vi "acquireAndDetectTest.vi"() -> ()   [LabVIEW 2024]
uses:
  src/elements/black-squircle-dropdown.ctl
  src/toolkit/modelParameters.ctl
  src/elements/black-squircle-ring.ctl
  <vilib>/Utility/error.llb/DialogType.ctl
  <vilib>/vision/driver/NI_Vision_Acquisition_Software.lvlib
  <resource>/objmgr/imaqdx.rc
  src/toolkit/transformCvToolkit.lvclass
panel:
  out "error status":string
  in  "update model":bool
  in  "res":T1 caption="Resolution:" items=["160x120 YUY2 30.00fps", "320x180 YUY2 30.00fps", "320x240 YUY2 30.00fps", "424x240 YUY2 30.00fps", "640x360 MJPG 30.00fps", "640x360 YUY2 30.00fps", "640x480 MJPG 30.00fps", "640x480 YUY2 30.00fps", "848x480 MJPG 30.00fps", "960x540 MJPG 30.00fps", "1280x720 MJPG 30.00fps"]
  in  "pause":bool
  in  "model params":T2={"conf"=0.25, "iou"=0.5, "model w"=1280, "model h"=736, "img w "=1280, "img h"=736} caption="Model Parameters"
  in  "classes":path caption="Class Definition Path"
  in  "model":path caption="Model Path"
  in  "cpu/gpu":enum32{"Item 0", "Item 1"}(radio)=enum."Item 1"
  in  "play":bool
  in  "cam":T3 caption="Camera:"
  out "img":T4(plugin-control)
  out "tot detect":i32 caption="Total Detections"
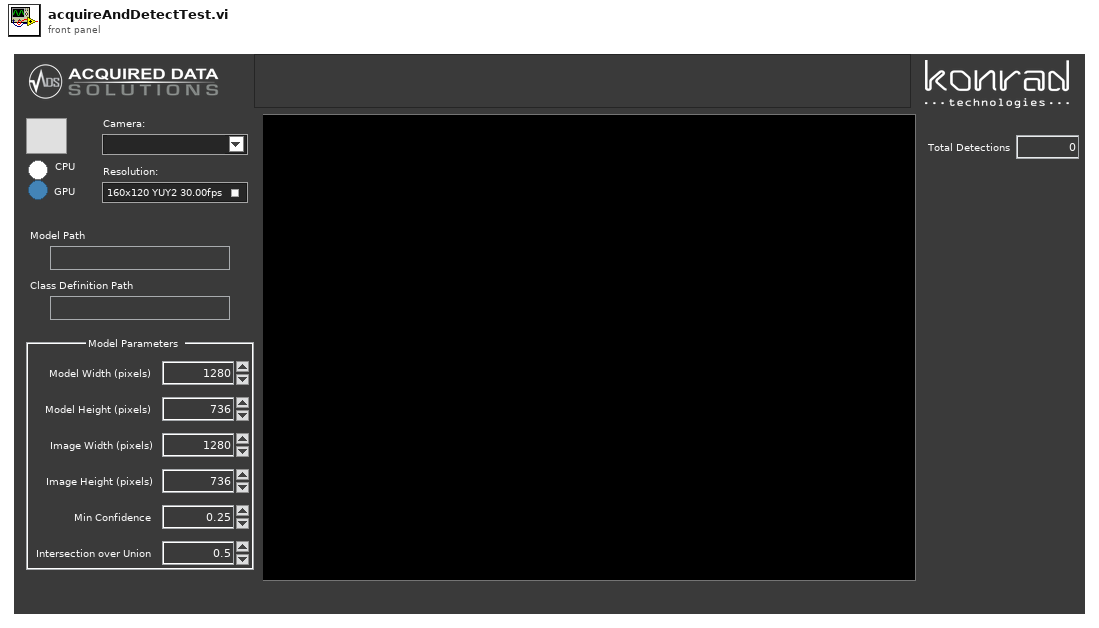
[diagram p1: front panel]
types:
  T1 = typedef "black-squircle-ring.ctl" = u16
  T2 = typedef "transformCvToolkit.lvclass/modelParameters.ctl" = cluster{"conf":dbl, "iou":dbl, "model w":i32, "model h":i32, "img w ":i32, "img h":i32}
  T3 = typedef "black-squircle-dropdown.ctl" = string
  T4 = typedef "IMAQ Image.ctl" = refnum<image>
  T5 = typedef "IMAQdx.ctl" = refnum<k21>
  T6 = typedef "DialogType.ctl" = u16
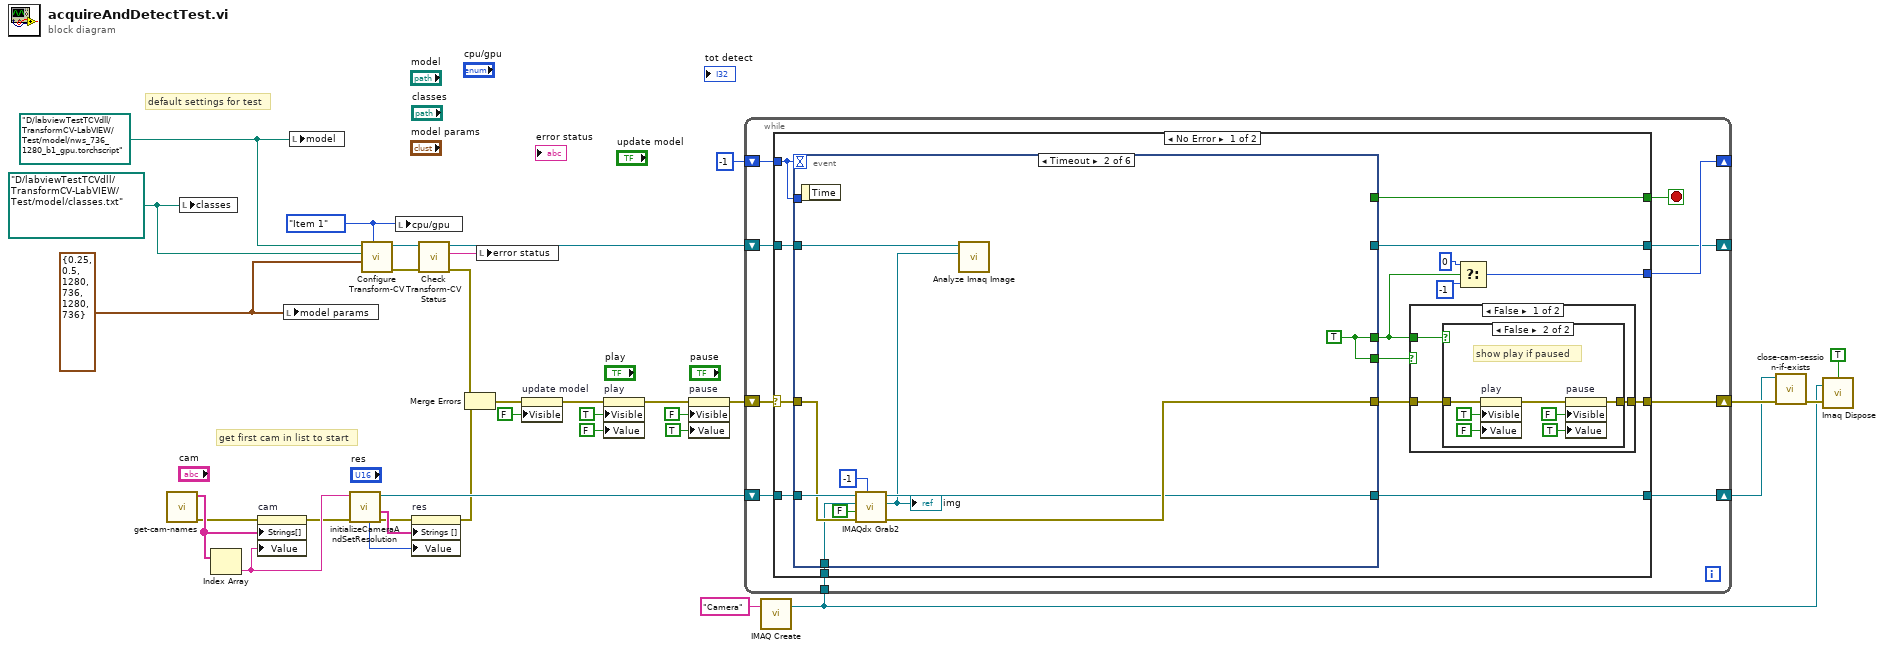
[diagram p0: block diagram]
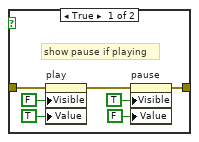
[diagram p2: hidden frame]
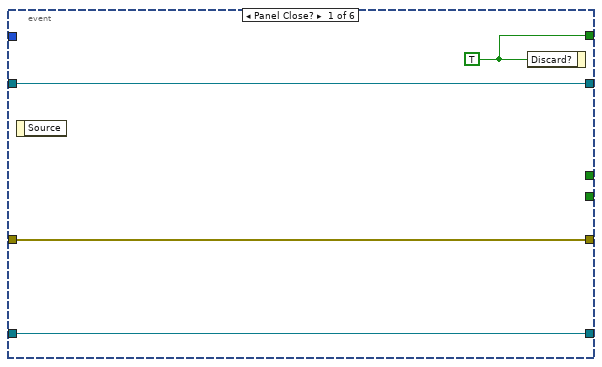
[diagram p4: hidden frame]
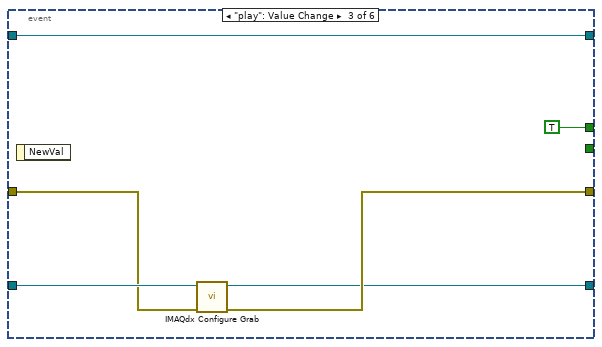
[diagram p5: hidden frame]
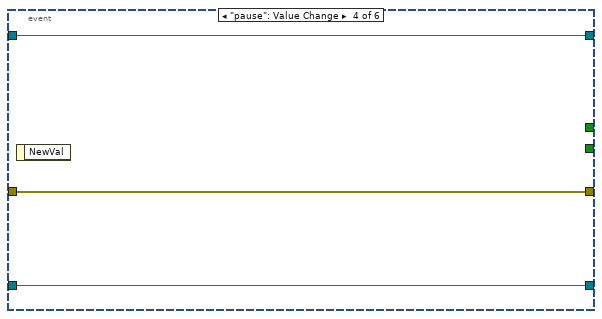
[diagram p6: hidden frame]
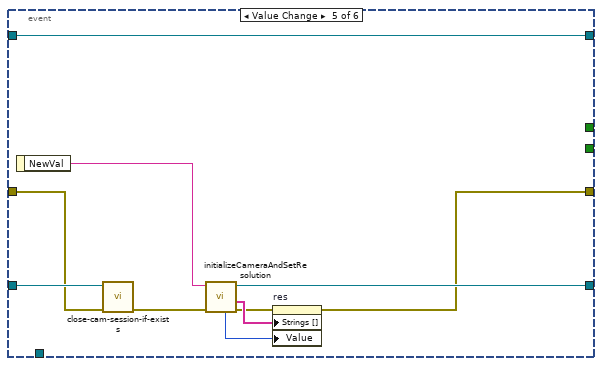
[diagram p7: hidden frame]
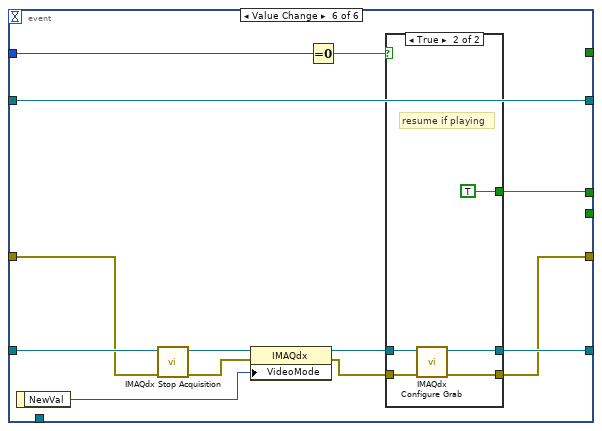
[diagram p8: hidden frame]
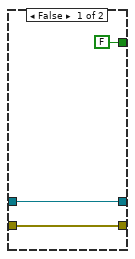
[diagram p9: hidden frame]
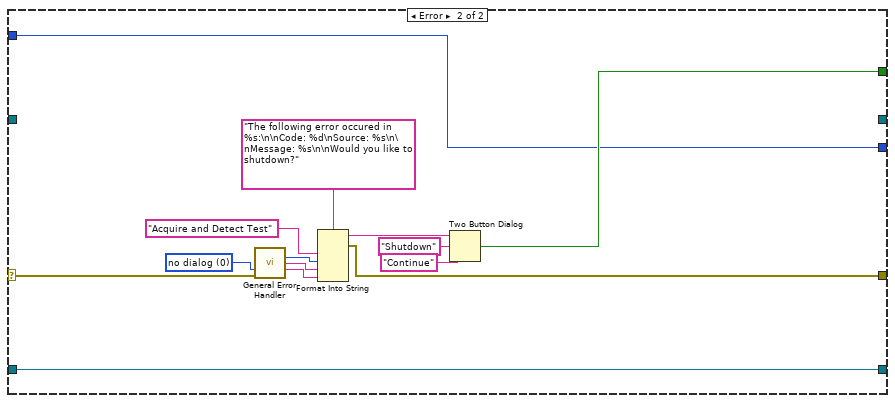
[diagram p10: hidden frame]
diagram:
  w6 = enum32{"Item 0", "Item 1"}."Item 1" ("cpu/gpu")
  w9 = T2 {"conf"=0.25, "iou"=0.5, "model w"=1280, "model h"=736, "img w "=1280, "img h"=736} ("model params")
  w10 = path "D:/labviewTestTCVdll/TransformCV-LabVIEW/Test/model/classes.txt" ("model")
  w11 = path "D:/labviewTestTCVdll/TransformCV-LabVIEW/Test/model/nws_736_1280_b1_gpu.torchscript" ("model")
  # "get first cam in list to start"
  # "default settings for test"
  n1 = call "get-cam-names.vi"() -> ("error out"=w12:errorcluster, "cam names"=w27:string[])  [unwired: 10 in]
  n2 = local write "classes"(w10) -> ()
  n3 = Index Array(array=w27) -> (element=w26:string)  [unwired: 1 in]
  n4 = property on="cam" class="CmbBox (strict)"(error in=w12, "Strings[]"=w27, "Value"=w26) -> (error out=w25:errorcluster)  [unwired: 1 in, 1 out]
  n5 = local write "model params"(w9) -> ()
  n6 = local write "model"(w11) -> ()
  n7 = call "initializeCameraAndSetResolution.vi"("error in"=w25, "seesion in"=w26) -> ("error out"=w22:errorcluster, "mode names"=w24:string[], "session out"=w21:T5, "current mode"=w23:u32)  [unwired: 5 in, 1 out]
  n8 = call "Configure Transform-CV.vi"("cpu/gpu"=w6, "model params"=w9, "classes"=w10, "model"=w11) -> ("error out"=w4:errorcluster, "transformCvToolkit out"=w5:refnum<class "transformCvToolkit.lvclass">)  [unwired: 5 in, 1 out]
  n9 = local write "cpu/gpu"(w6) -> ()
  n10 = property on="res" class="Ring (strict)"(error in=w22, "Strings []"=w24, "Value"=w23) -> (error out=w8:errorcluster)  [unwired: 1 in, 1 out]
  n11 = call "Check Transform-CV Status.vi"("error in (no error)"=w4, "transformCvToolkit in"=w5) -> ("error out"=w3:errorcluster, "status"=w1:string, "transformCvToolkit out"=w2:refnum<class "transformCvToolkit.lvclass">)  [unwired: 7 in]
  n12 = Merge Errors(w3, w8) -> (w7:errorcluster)
  n13 = local write "error status"(w1) -> ()
  n14 = property on="update model" class="Bool"(error in=w7, "Visible"=FALSE) -> (error out=w14:errorcluster)  [unwired: 1 in, 1 out]
  n15 = property on="play" class="Bool (strict)"(error in=w14, "Visible"=TRUE, "Value"=FALSE ("play")) -> (error out=w32:errorcluster)  [unwired: 1 in, 1 out]
  n16 = property on="pause" class="Bool (strict)"(error in=w32, "Visible"=FALSE, "Value"=TRUE ("Visible")) -> (error out=w33:errorcluster)  [unwired: 1 in, 1 out]
  n17 = call "IMAQ Create"("Image Name"="Camera") -> ("New Image"=w15:T4)  [unwired: 4 in, 1 out]
  n18 = while {
    shift-right: [w44] -> w20
    shift-left: w33 -> [w43]
    shift-right: [w40] -> _
    shift-left: -1 -> [w41]
    shift-right: [w38] -> w19
    shift-left: w21 -> [w39]
    tunnel: w15 -> [w37]
    shift-right: [w35] -> _
    shift-left: w2 -> [w36]
    stop <- w42 stop-if-true
    n19 = case shown="No Error" w43 {
      selector: w43 -> [w59 w137]
      tunnel: [w53 w135] -> w44
      tunnel: [w58 w136] -> w42
      tunnel: w41 -> [w47 w133]
      tunnel: [w55 w133] -> w40
      tunnel: w39 -> [w50 w132]
      tunnel: [w49 w132] -> w38
      tunnel: w37 -> [w48 _]
      tunnel: w36 -> [w46 _]
      tunnel: [w45 _] -> w35
      frame No Error {
        n20 = event shown="[1] Timeout" {
          selector: _ -> [_ _ _ _ _ _]
          dyn-events: _ -> [_ _ _ _ _ _]
          timeout: w47 -> [_ _ _ _ _ _]
          tunnel: w59 -> [w81 w87 w95 w100 w104 w120]
          tunnel: [w79 _ _ _ _ _] -> w58
          tunnel: [w81 w86 w94 w100 w102 w113] -> w54
          tunnel: [_ w91 TRUE ("s") _ _ w112] -> w52
          tunnel: [_ w91 _ _ _ _] -> w51
          tunnel: w50 -> [w80 w88 w96 w99 w105 w122]
          tunnel: [w80 w85 w93 w99 w109 w114] -> w49
          tunnel: w48 -> [_ w84 _ _ _ _]
          tunnel: w47 -> [_ _ _ _ _ w118]
          tunnel: w46 -> [w78 w83 w92 w98 w101 w111]
          tunnel: [w78 _ w92 w98 w101 w111] -> w45
          event Panel Close? {
            w79 = TRUE ("Discard?")
            n21 = event-data() -> ()  [unwired: 1 in, 1 out]
            n22 = event-data("Discard?"=w79) -> ()  [unwired: 1 in, 1 out]
          }
          event Timeout {
            w91 = TRUE ("s")
            n23 = event-data() -> ()  [unwired: 1 in, 1 out]
            n24 = call <vilib>:"IMAQdx Grab2.vi"("Timeout (ms)"=-1, "error in"=w87, "Wait for Next Buffer? (Yes)"=FALSE, "Image In"=w84, "Session In"=w88) -> ("error out"=w86:errorcluster, "Image Out"=w82:T4, "Session Out"=w85:T5)  [unwired: 3 in, 1 out]
            "img" <- w82
            n25 = call "Analyze Imaq Image.vi"("imaq image ref"=w82, "transformCvToolkit in"=w83) -> ()  [unwired: 8 in, 2 out]
          }
          event "play": Value Change {
            n26 = event-data() -> ()  [unwired: 1 in, 1 out]
            n27 = call <vilib>:"IMAQdx Configure Grab.vi"("error in"=w95, "Session In"=w96) -> ("error out"=w94:errorcluster, "Session Out"=w93:T5)  [unwired: 8 in]
          }
          event "pause": Value Change {
            n28 = event-data() -> ()  [unwired: 1 in, 1 out]
          }
          event Value Change {
            n29 = event-data() -> ("NewVal"=w110:T3)  [unwired: 1 in]
            n30 = call "close-cam-session-if-exists.vi"("error in (no error)"=w104, "cam in"=w105) -> ("error out"=w103:errorcluster)  [unwired: 9 in]
            n31 = call "initializeCameraAndSetResolution.vi"("error in"=w103, "seesion in"=w110) -> ("error out"=w107:errorcluster, "mode names"=w108:string[], "session out"=w109:T5, "current mode"=w106:u32)  [unwired: 5 in, 1 out]
            n32 = property on="res" class="Ring (strict)"(error in=w107, "Strings []"=w108, "Value"=w106) -> (error out=w102:errorcluster)  [unwired: 1 in, 1 out]
          }
          event Value Change {
            n33 = event-data() -> ("NewVal"=w123:T1)  [unwired: 1 in]
            n34 = call <vilib>:"IMAQdx Stop Acquisition.vi"("error in"=w120, "Session In"=w122) -> ("error out"=w119:errorcluster, "Session Out"=w121:T5)  [unwired: 8 in]
            n35 = property class="IMAQdx"(reference=w121, error in=w119, "VideoMode"=w123) -> (reference out=w116:T5, error out=w115:errorcluster)
            n36 = Equal To 0?(x=w118) -> (x = 0?=w117:bool)
            n37 = case shown="True" w117 {
              tunnel: w116 -> [w125 w131]
              tunnel: w115 -> [w124 w130]
              tunnel: [w125 w129] -> w114
              tunnel: [w124 w128] -> w113
              tunnel: [FALSE ("s") TRUE ("s")] -> w112
              frame False {
              }
              frame True {
                # "resume if playing"
                n38 = call <vilib>:"IMAQdx Configure Grab.vi"("error in"=w130, "Session In"=w131) -> ("error out"=w128:errorcluster, "Session Out"=w129:T5)  [unwired: 8 in]
              }
            }
          }
        }
        n39 = case shown="False" w51 {
          tunnel: w54 -> [w62 w77]
          tunnel: [w61 w77] -> w53
          tunnel: w52 -> [w60 _]
          frame False {
            n40 = case shown="False" w60 {
              tunnel: w62 -> [w64 w71]
              tunnel: [w63 w70] -> w61
              frame True {
                # "show pause if playing"
                n41 = property on="play" class="Bool (strict)"(error in=w64, "Visible"=FALSE, "Value"=TRUE ("play")) -> (error out=w66:errorcluster)  [unwired: 1 in, 1 out]
                n42 = property on="pause" class="Bool (strict)"(error in=w66, "Visible"=TRUE, "Value"=FALSE ("Visible")) -> (error out=w63:errorcluster)  [unwired: 1 in, 1 out]
              }
              frame False {
                # "show play if paused"
                n43 = property on="play" class="Bool (strict)"(error in=w71, "Visible"=TRUE, "Value"=FALSE ("play")) -> (error out=w73:errorcluster)  [unwired: 1 in, 1 out]
                n44 = property on="pause" class="Bool (strict)"(error in=w73, "Visible"=FALSE, "Value"=TRUE ("Visible")) -> (error out=w70:errorcluster)  [unwired: 1 in, 1 out]
              }
            }
          }
          frame True {
            # "don't waste time on update if running continuous acquisition"
          }
        }
        n45 = Select(t=0, s=w52, f=-1) -> (s? t:f=w55:i32)
      }
      frame Error {
        w145 = T6 0 items=["no dialog", "OK message", "continue or stop message", "OK message + warnings", "continue/stop + warnings"] ("type of dialog (OK msg:1)")
        n46 = call <vilib>:"General Error Handler.vi"("type of dialog (OK msg:1)"=w145, "error in (no error)"=w137) -> ("code out"=w138:i32, "source out"=w140:string, "message"=w141:string)  [unwired: 9 in, 2 out]
        n47 = Format Into String(format string="The following error occured in %s:\n\nCode: %d\nSource: %s\n\nMessage: %s\n\nWould you like to shutdown?", "Acquire and Detect Test" ("input 1"), w138, w140, w141) -> (resulting string=w142:string, error out=w135:errorcluster)  [unwired: 2 in]
        n48 = Two Button Dialog(message=w142, 1:"Continue" ("F button name (\"Cancel\")"), 2:"Shutdown" ("T button name (\"OK\")")) -> (T button?=w136:bool)
      }
    }
  }
  n49 = call "close-cam-session-if-exists.vi"("error in (no error)"=w20, "cam in"=w19) -> ("error out"=w17:errorcluster)  [unwired: 9 in]
  n50 = call "Imaq Dispose"("All Images? (No)"=TRUE, "Image"=w15, "error in (no error)"=w17) -> ()  [unwired: 3 in, 1 out]
